vi "Calculate Phase Calibration Constants.vi"() -> ()   [LabVIEW 2015]
doc: "Calculates the phase difference between the the LO sharing channel and all other channels by injecting a common tone into all the receiving channels. This is done over multiple runs to provide the mean phase differences between channels at the requested carrier frequencies."
uses:
  <vilib>/Analysis/NI_AALBase.lvlib
panel:
  out "ch3-ch2":dbl
  out "ch2-ch2":dbl
  out "ch1-ch2":dbl
  out "ch0-ch2":dbl
  out "Std Dev of Phase Offsets":T1
  out "Mean Phase Offsets":T1
  in  "Carrier Frequency":dbl=900000000.0 format="%#_6p"
  out "error out":errorcluster
  in  "Tx Device Name":refnum<k15>="192.168.10.2"
  in  "Rx Device Name":refnum<k15>="192.168.10.3"
  in  "Number of Averages":i32=5
  # "Phase Calibration Constants"
  # "ch0-ch2"
  # "ch1-ch2"
  # "ch2-ch2"
  # "ch3-ch2"
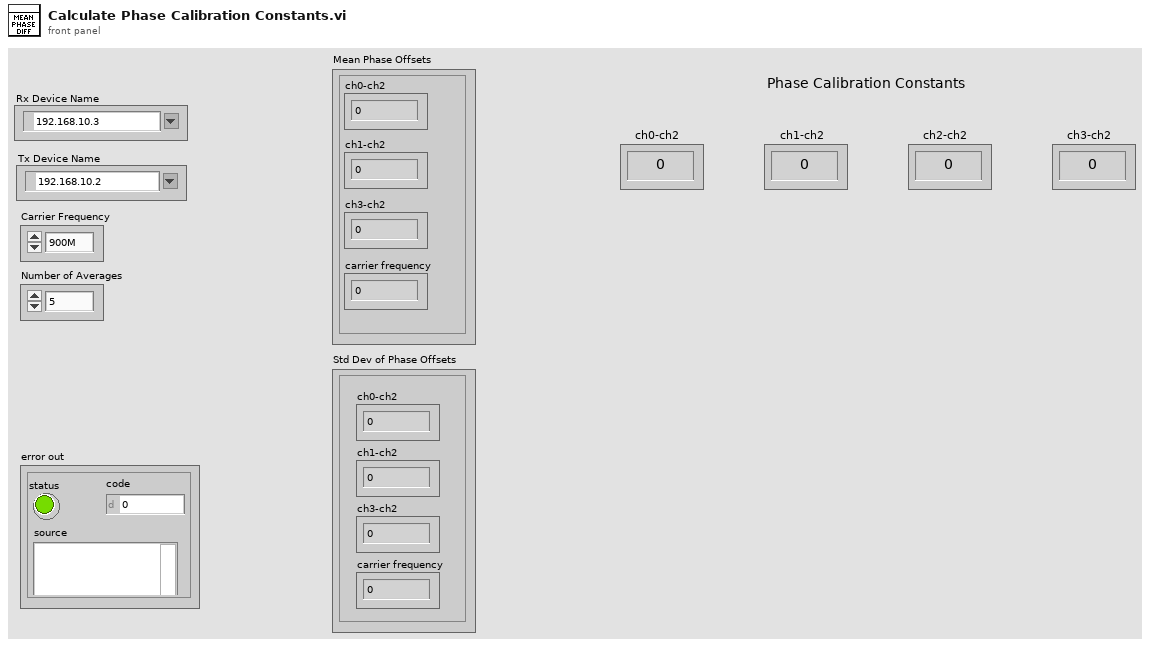
[diagram p1: front panel]
types:
  T1 = cluster{"ch0-ch2":dbl, "ch1-ch2":dbl, "ch3-ch2":dbl, "carrier frequency":dbl}
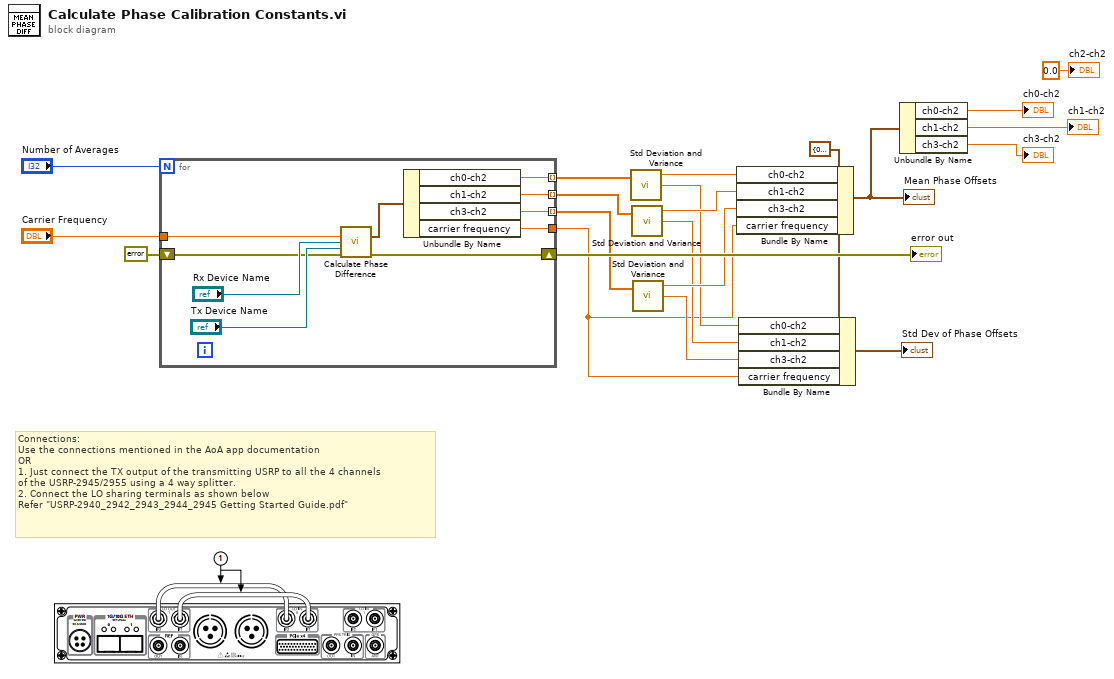
[diagram p0: block diagram]
diagram:
  w8 = T1 {"ch0-ch2"=0.0, "ch1-ch2"=0.0, "ch3-ch2"=0.0, "carrier frequency"=0.0} ("input cluster")
  # "Connections:\nUse the connections mentioned in the AoA app documentation\nOR\n1. Just connect the TX output of the transmitting USRP to all the 4 channels\nof the USRP-2945/2955 using a 4 way splitter.\n2. Connect the LO sharing terminals as shown below\nRefer \"USRP-2940_2942_2943_2944_2945 Getting Started Guide.pdf\""
  n1 = for {
    N: "Number of Averages" -> [_]
    tunnel: [w31] -> w18 mode=indexing
    tunnel: [w30] -> w17 mode=indexing
    tunnel: [w29] -> w16 mode=indexing
    tunnel: [w28] -> w9
    shift-right: [w25] -> w21
    shift-left: errorcluster {"status"=FALSE, "code"=0, "source"=""} ("error out") -> [w24]
    tunnel: "Carrier Frequency" -> [w22]
    n2 = call "Calculate Phase Difference.vi"("Carrier Frequency"=w22, "Rx Device Name"="Rx Device Name", "Tx Device Name"="Tx Device Name", "error in"=w24) -> ("Phase Differences"=w23:T1, "error out"=w25:errorcluster)  [unwired: 10 in]
    n3 = Unbundle By Name(w23) -> ("ch0-ch2"=w31:dbl, "ch1-ch2"=w30:dbl, "ch3-ch2"=w29:dbl, "carrier frequency"=w28:dbl)
  }
  "error out" <- w21
  n4 = call <vilib>:"Std Deviation and Variance.vi"("X"=w18) -> ("mean"=w15:dbl, "standard deviation"=w12:dbl)  [unwired: 1 in, 1 out]
  n5 = call <vilib>:"Std Deviation and Variance.vi"("X"=w17) -> ("mean"=w14:dbl, "standard deviation"=w11:dbl)  [unwired: 1 in, 1 out]
  n6 = call <vilib>:"Std Deviation and Variance.vi"("X"=w16) -> ("mean"=w13:dbl, "standard deviation"=w10:dbl)  [unwired: 1 in, 1 out]
  n7 = Bundle By Name(cluster=w8, "ch0-ch2"=w15, "ch1-ch2"=w14, "ch3-ch2"=w13, "carrier frequency"=w9) -> (w5:T1)
  "Mean Phase Offsets" <- w5
  n8 = Bundle By Name(cluster=w8, "ch0-ch2"=w12, "ch1-ch2"=w11, "ch3-ch2"=w10, "carrier frequency"=w9) -> (→"Std Dev of Phase Offsets":T1)
  n9 = Unbundle By Name(w5) -> ("ch0-ch2"=→"ch0-ch2":dbl, "ch1-ch2"=→"ch1-ch2":dbl, "ch3-ch2"=→"ch3-ch2":dbl)
  "ch2-ch2" <- 0.0 ("ch2-ch2")
